vi "Catch_screw(start_side).vi"(6 "向哪校正":T1(ring)=enum."right", 7 "櫃子在哪?":enum16{"前面", "左邊", "右邊"}(ring), 8 "Error In":errorcluster) -> (0 "Error Out":errorcluster, 3 "it2(nut)":string)   [LabVIEW 2019]
uses:
  WSCbot_V3_Toolkit.lvlibp/WSCBOTV3_Toolkit/IO/LowLevel/PulseCounter.ctl
  WSCbot_V3_Toolkit.lvlibp
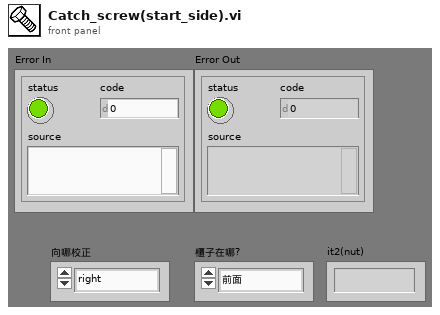
[diagram p1: front panel]
types:
  T1 = enum16{"Right_up", "Right_down", "Left_down", "Left_up", "left", "right", "up", "down"}
  T2 = typedef "WSCbot_V3_Toolkit.lvlibp/PulseCounter.ctl" = enum16{"CH1", "CH2", "CH3", "CH4", "CH5"}
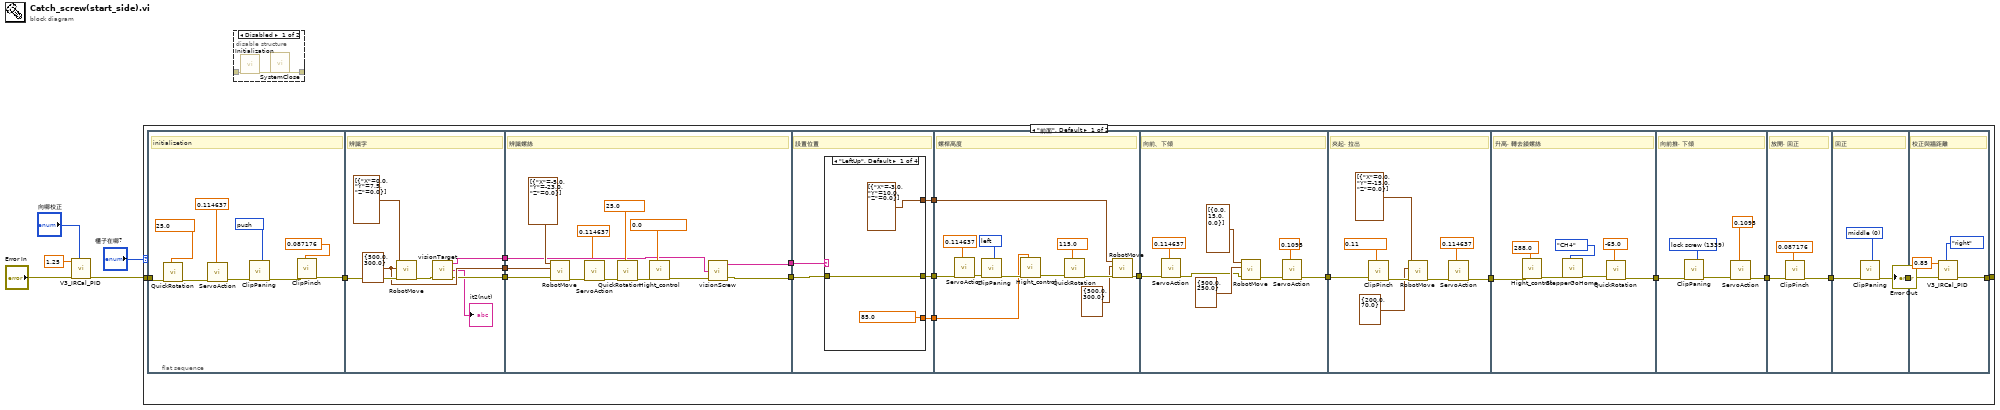
[diagram p0: block diagram]
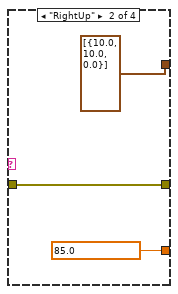
[diagram p2: hidden frame]
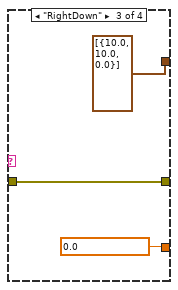
[diagram p3: hidden frame]
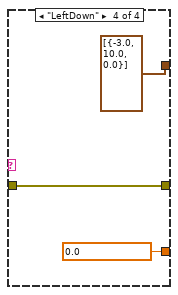
[diagram p4: hidden frame]
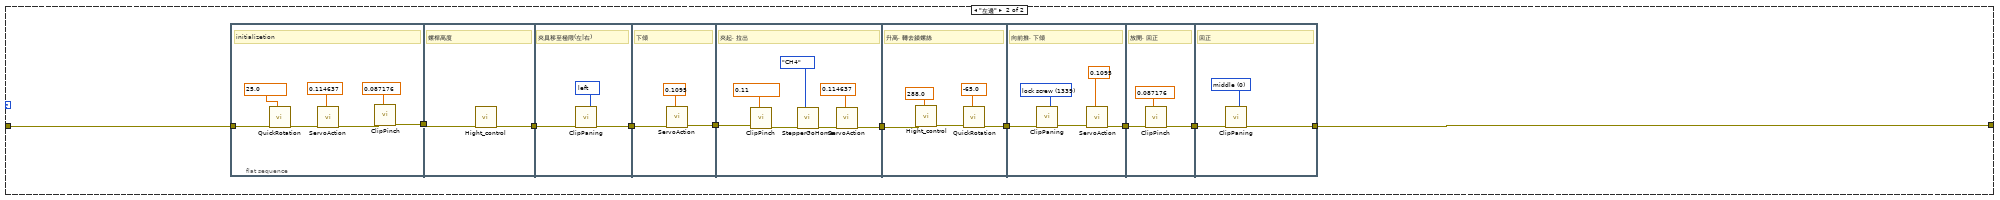
[diagram p5: hidden frame]
diagram:
  n1 = call "V3_IRCal_PID.vi"("Direction"="向哪校正", "Error In"="Error In", "X_distance(V)"=1.25) -> ("Error Out"=w4:errorcluster)  [unwired: 7 in, 1 out]
  n2 = case shown="\"前面\", Default" "櫃子在哪?" {
    tunnel: [w8 w122] -> w6
    tunnel: w4 -> [w19 w121]
    frame "前面", Default {
      n3 = flat-sequence {
        tunnel: [w28] -> w18
        tunnel: w19 -> [w27]
        tunnel: w18 -> [w39]
        tunnel: [w38] -> w17
        tunnel: [w37] -> w16
        tunnel: [w35] -> w15
        tunnel: w17 -> [w45]
        tunnel: w16 -> [w43]
        tunnel: w15 -> [w47]
        tunnel: [w44] -> w13
        tunnel: [w42] -> w12
        tunnel: w13 -> [w58]
        tunnel: w12 -> [w57]
        tunnel: [w56] -> w11
        tunnel: [w55] -> w10
        tunnel: [w54] -> w7
        tunnel: [w80] -> w14
        tunnel: w11 -> [w79]
        tunnel: w10 -> [w77]
        tunnel: w7 -> [w71]
        tunnel: [w90] -> w24
        tunnel: w14 -> [w84]
        tunnel: [w96] -> w23
        tunnel: w24 -> [w97]
        tunnel: w23 -> [w103]
        tunnel: [w104] -> w22
        tunnel: w22 -> [w110]
        tunnel: [w106] -> w21
        tunnel: w21 -> [w113]
        tunnel: [w111] -> w20
        tunnel: w20 -> [w115]
        tunnel: [w114] -> w9
        tunnel: w9 -> [w120]
        tunnel: [w119] -> w8
        frame #0 {
          w25 = 0.114637 items=["up"=0.107, "lock_up"=0.111528, "up_up"=0.114637, "down"=0.073446, "back"=0.037435, "back_back"=0.035] ("face_dir")
          w26 = -2700 items=["left"=2250, "right"=-3500, "lock screw"=1345, "lock_nut"=1167, "push"=-2700, "middle"=0] ("location")
          w32 = 25.0 items=["Forward"=25.0, "Right"=115.0, "Left"=-65.0] ("螺桿面向")
          w31 = 0.087176 items=["pinch_up"=0.11, "release"=0.087176] ("pinch?")
          # "initializetion"
          n4 = call "QuickRotation.vi"("螺桿面向"=w32, "Error In"=w27) -> ("Error Out"=w33:errorcluster)  [unwired: 9 in]
          n5 = call "ServoAction.vi"("face_dir"=w25, "Error In"=w33) -> ("Error Out"=w29:errorcluster)  [unwired: 9 in]
          n6 = call "ClipPaning.vi"("Error In"=w29, "location"=w26) -> ("Error Out"=w30:errorcluster)  [unwired: 8 in]
          n7 = call "ClipPinch.vi"("pinch?"=w31, "Error In"=w30) -> ("Error Out"=w28:errorcluster)  [unwired: 9 in]
        }
        frame #1 {
          w37 = cluster{dbl, dbl} {500.0, 300.0} ("Speed/ACC")
          # "辨識字"
          n8 = call "RobotMove.vi"("error in (no error)"=w39, "Speed/ACC"=w37, "XYZ"=cluster{"X":dbl, "Y":dbl, "Z":dbl}[] [{"X"=0.0, "Y"=7.5, "Z"=0.0}]) -> ("error out"=w36:errorcluster)  [unwired: 8 in]
          n9 = call "visionTarget.vi"("Error In"=w36) -> ("Error Out"=w35:errorcluster, "it2(nut)"=→"it2(nut)":string, "it1(screw)"=w38:string)  [unwired: 2 in]
        }
        frame #2 {
          w41 = 0.114637 items=["up"=0.107, "lock_up"=0.111528, "up_up"=0.114637, "down"=0.073446, "back"=0.037435, "back_back"=0.035] ("face_dir")
          w48 = 0.0 items=["物料櫃第一格"=0.0, "物料櫃第二格"=78.0, "螺帽夾取高度"=128.0, "螺帽瞄準"=250.0, "最高"=288.0] ("螺桿高度")
          w50 = 25.0 items=["Forward"=25.0, "Right"=115.0, "Left"=-65.0] ("螺桿面向")
          # "辨識螺絲"
          n10 = call "RobotMove.vi"("error in (no error)"=w47, "Speed/ACC"=w43, "XYZ"=cluster{"X":dbl, "Y":dbl, "Z":dbl}[] [{"X"=-5.0, "Y"=-23.0, "Z"=0.0}]) -> ("error out"=w52:errorcluster)  [unwired: 8 in]
          n11 = call "ServoAction.vi"("face_dir"=w41, "Error In"=w52) -> ("Error Out"=w51:errorcluster)  [unwired: 9 in]
          n12 = call "QuickRotation.vi"("螺桿面向"=w50, "Error In"=w51) -> ("Error Out"=w49:errorcluster)  [unwired: 9 in]
          n13 = call "Hight_control.vi"("螺桿高度"=w48, "Error In"=w49) -> ("Error Out"=w46:errorcluster)  [unwired: 9 in]
          n14 = call "visionScrew.vi"("Error In"=w46, "Aim_Color"=w45) -> ("Error Out"=w42:errorcluster, "Position"=w44:string)  [unwired: 2 in]
        }
        frame #3 {
          # "設置位置"
          n15 = case shown="\"LeftUp\", Default" w58 {
            tunnel: w57 -> [w60 w63 w66 w69]
            tunnel: [cluster{"X":dbl, "Y":dbl, "Z":dbl}[] [{"X"=-3.0, "Y"=10.0, "Z"=0.0}] ("XYZ") cluster{"X":dbl, "Y":dbl, "Z":dbl}[] [{"X"=10.0, "Y"=10.0, "Z"=0.0}] ("XYZ") cluster{"X":dbl, "Y":dbl, "Z":dbl}[] [{"X"=10.0, "Y"=10.0, "Z"=0.0}] ("XYZ") cluster{"X":dbl, "Y":dbl, "Z":dbl}[] [{"X"=-3.0, "Y"=10.0, "Z"=0.0}] ("XYZ")] -> w56
            tunnel: [w60 w63 w66 w69] -> w55
            tunnel: [w59 w62 w65 w68] -> w54
            frame "LeftUp", Default {
              w59 = 85.0 items=["物料櫃第一格"=0.0, "物料櫃第二格"=85.0, "螺帽夾取高度"=128.0, "螺帽瞄準"=250.0, "最高"=288.0] ("螺桿高度")
            }
            frame "RightUp" {
              w62 = 85.0 items=["物料櫃第一格"=0.0, "物料櫃第二格"=85.0, "螺帽夾取高度"=128.0, "螺帽瞄準"=250.0, "最高"=288.0] ("螺桿高度")
            }
            frame "RightDown" {
              w65 = 0.0 items=["物料櫃第一格"=0.0, "物料櫃第二格"=85.0, "螺帽夾取高度"=128.0, "螺帽瞄準"=250.0, "最高"=288.0] ("螺桿高度")
            }
            frame "LeftDown" {
              w68 = 0.0 items=["物料櫃第一格"=0.0, "物料櫃第二格"=85.0, "螺帽夾取高度"=128.0, "螺帽瞄準"=250.0, "最高"=288.0] ("螺桿高度")
            }
          }
        }
        frame #4 {
          w72 = 0.114637 items=["up"=0.107, "lock_up"=0.111528, "up_up"=0.114637, "down"=0.073446, "back"=0.037435, "back_back"=0.035] ("face_dir")
          w82 = 2100 items=["left"=2100, "right"=-3500, "lock screw"=1345, "lock_nut"=1167, "middle"=0] ("location")
          w75 = 115.0 items=["Forward"=25.0, "Right"=115.0, "Left"=-65.0] ("螺桿面向")
          # "螺桿高度"
          n16 = call "ServoAction.vi"("face_dir"=w72, "Error In"=w77) -> ("Error Out"=w76:errorcluster)  [unwired: 9 in]
          n17 = call "ClipPaning.vi"("Error In"=w76, "location"=w82) -> ("Error Out"=w74:errorcluster)  [unwired: 8 in]
          n18 = call "Hight_control.vi"("螺桿高度"=w71, "Error In"=w74) -> ("Error Out"=w73:errorcluster)  [unwired: 9 in]
          n19 = call "QuickRotation.vi"("螺桿面向"=w75, "Error In"=w73) -> ("Error Out"=w81:errorcluster)  [unwired: 9 in]
          n20 = call "RobotMove.vi"("error in (no error)"=w81, "Speed/ACC"=cluster{dbl, dbl} {500.0, 300.0}, "XYZ"=w79) -> ("error out"=w80:errorcluster)  [unwired: 8 in]
        }
        frame #5 {
          w85 = 0.114637 items=["up"=0.1095, "up_up"=0.114637, "down"=0.073446, "back"=0.037435, "back_back"=0.035] ("face_dir")
          w89 = 0.1095 items=["up"=0.1095, "up_up"=0.114637, "down"=0.073446, "back"=0.037435, "back_back"=0.035] ("face_dir")
          # "向前、下傾"
          n21 = call "ServoAction.vi"("face_dir"=w85, "Error In"=w84) -> ("Error Out"=w83:errorcluster)  [unwired: 9 in]
          n22 = call "RobotMove.vi"("error in (no error)"=w83, "Speed/ACC"=cluster{dbl, dbl} {500.0, 250.0}, "XYZ"=cluster{"X":dbl, "Y":dbl, "Z":dbl}[] [{"X"=0.0, "Y"=15.0, "Z"=0.0}]) -> ("error out"=w88:errorcluster)  [unwired: 8 in]
          n23 = call "ServoAction.vi"("face_dir"=w89, "Error In"=w88) -> ("Error Out"=w90:errorcluster)  [unwired: 9 in]
        }
        frame #6 {
          w95 = 0.114637 items=["up"=0.1095, "up_up"=0.114637, "down"=0.073446, "back"=0.037435, "back_back"=0.035] ("face_dir")
          w98 = 0.11 items=["pinch_up"=0.11, "release"=0.087176] ("pinch?")
          # "夾起, 拉出"
          n24 = call "ClipPinch.vi"("pinch?"=w98, "Error In"=w97) -> ("Error Out"=w94:errorcluster)  [unwired: 9 in]
          n25 = call "RobotMove.vi"("error in (no error)"=w94, "Speed/ACC"=cluster{dbl, dbl} {200.0, 70.0}, "XYZ"=cluster{"X":dbl, "Y":dbl, "Z":dbl}[] [{"X"=0.0, "Y"=-15.0, "Z"=0.0}]) -> ("error out"=w93:errorcluster)  [unwired: 8 in]
          n26 = call "ServoAction.vi"("face_dir"=w95, "Error In"=w93) -> ("Error Out"=w96:errorcluster)  [unwired: 9 in]
        }
        frame #7 {
          w102 = 288.0 items=["物料櫃第一格"=0.0, "物料櫃第二格"=78.0, "螺帽夾取高度"=128.0, "螺帽瞄準"=250.0, "最高"=288.0] ("螺桿高度")
          w105 = -65.0 items=["Forward"=25.0, "Right"=115.0, "Left"=-65.0] ("螺桿面向")
          # "升高, 轉去鎖螺絲"
          n27 = call "Hight_control.vi"("螺桿高度"=w102, "Error In"=w103) -> ("Error Out"=w100:errorcluster)  [unwired: 9 in]
          n28 = call "StepperGoHome.vi"("PulseCounterChanel"=PulseCounter."CH4", "Error In"=w100) -> ("Error Out"=w99:errorcluster)  [unwired: 7 in, 2 out]
          n29 = call "QuickRotation.vi"("螺桿面向"=w105, "Error In"=w99) -> ("Error Out"=w104:errorcluster)  [unwired: 9 in]
        }
        frame #8 {
          w107 = 0.1095 items=["up"=0.1095, "up_up"=0.114637, "down"=0.073446, "back"=0.037435, "back_back"=0.035] ("face_dir")
          w109 = 1339 items=["left"=2100, "right"=-3500, "lock screw"=1339, "middle"=0] ("location")
          # "向前推, 下傾"
          n30 = call "ClipPaning.vi"("Error In"=w110, "location"=w109) -> ("Error Out"=w108:errorcluster)  [unwired: 8 in]
          n31 = call "ServoAction.vi"("face_dir"=w107, "Error In"=w108) -> ("Error Out"=w106:errorcluster)  [unwired: 9 in]
        }
        frame #9 {
          w112 = 0.087176 items=["pinch_up"=0.11, "release"=0.087176] ("pinch?")
          # "放開, 回正"
          n32 = call "ClipPinch.vi"("pinch?"=w112, "Error In"=w113) -> ("Error Out"=w111:errorcluster)  [unwired: 9 in]
        }
        frame #10 {
          w116 = 0 items=["left"=2100, "right"=-3500, "lock screw"=1339, "middle"=0] ("location")
          # "回正"
          n33 = call "ClipPaning.vi"("Error In"=w115, "location"=w116) -> ("Error Out"=w114:errorcluster)  [unwired: 8 in]
        }
        frame #11 {
          # "校正與牆距離"
          n34 = call "V3_IRCal_PID.vi"("Direction"=T1."right", "Error In"=w120, "X_distance(V)"=0.85) -> ("Error Out"=w119:errorcluster)  [unwired: 7 in, 1 out]
        }
      }
    }
    frame "左邊" {
      n35 = flat-sequence {
        tunnel: [w134] -> w130
        tunnel: w121 -> [w132]
        tunnel: w130 -> [w139]
        tunnel: [w138] -> w129
        tunnel: [w142] -> w128
        tunnel: w129 -> [w140]
        tunnel: w128 -> [w144]
        tunnel: [w145] -> w127
        tunnel: [w147] -> w126
        tunnel: w127 -> [w149]
        tunnel: w126 -> [w155]
        tunnel: [w156] -> w125
        tunnel: w125 -> [w162]
        tunnel: [w158] -> w124
        tunnel: w124 -> [w165]
        tunnel: [w163] -> w123
        tunnel: w123 -> [w167]
        tunnel: [w166] -> w122
        frame #0 {
          w131 = 25.0 items=["Forward"=25.0, "Right"=115.0, "Left"=-65.0] ("螺桿面向")
          w136 = 0.087176 items=["pinch_up"=0.11, "release"=0.087176] ("pinch?")
          w137 = 0.114637 items=["up"=0.1095, "up_up"=0.114637, "down"=0.073446, "back"=0.037435, "back_back"=0.035] ("face_dir")
          # "initializetion"
          n36 = call "QuickRotation.vi"("螺桿面向"=w131, "Error In"=w132) -> ("Error Out"=w133:errorcluster)  [unwired: 9 in]
          n37 = call "ServoAction.vi"("face_dir"=w137, "Error In"=w133) -> ("Error Out"=w135:errorcluster)  [unwired: 9 in]
          n38 = call "ClipPinch.vi"("pinch?"=w136, "Error In"=w135) -> ("Error Out"=w134:errorcluster)  [unwired: 9 in]
        }
        frame #1 {
          # "螺桿高度"
          n39 = call "Hight_control.vi"("Error In"=w139) -> ("Error Out"=w138:errorcluster)  [unwired: 10 in]
        }
        frame #2 {
          w141 = 2100 items=["left"=2100, "right"=-3500, "lock screw"=1339, "middle"=0] ("location")
          # "夾具移至極限(左|右)"
          n40 = call "ClipPaning.vi"("Error In"=w140, "location"=w141) -> ("Error Out"=w142:errorcluster)  [unwired: 8 in]
        }
        frame #3 {
          w143 = 0.1095 items=["up"=0.1095, "up_up"=0.114637, "down"=0.073446, "back"=0.037435, "back_back"=0.035] ("face_dir")
          # "下傾"
          n41 = call "ServoAction.vi"("face_dir"=w143, "Error In"=w144) -> ("Error Out"=w145:errorcluster)  [unwired: 9 in]
        }
        frame #4 {
          w146 = 0.114637 items=["up"=0.1095, "up_up"=0.114637, "down"=0.073446, "back"=0.037435, "back_back"=0.035] ("face_dir")
          w152 = 0.11 items=["pinch_up"=0.11, "release"=0.087176] ("pinch?")
          # "夾起, 拉出"
          n42 = call "ClipPinch.vi"("pinch?"=w152, "Error In"=w149) -> ("Error Out"=w151:errorcluster)  [unwired: 9 in]
          n43 = call "StepperGoHome.vi"("PulseCounterChanel"=PulseCounter."CH4", "Error In"=w151) -> ("Error Out"=w148:errorcluster)  [unwired: 7 in, 2 out]
          n44 = call "ServoAction.vi"("face_dir"=w146, "Error In"=w148) -> ("Error Out"=w147:errorcluster)  [unwired: 9 in]
        }
        frame #5 {
          w153 = 288.0 items=["物料櫃第一格"=0.0, "物料櫃第二格"=78.0, "螺帽夾取高度"=128.0, "螺帽瞄準"=250.0, "最高"=288.0] ("螺桿高度")
          w157 = -65.0 items=["Forward"=25.0, "Right"=115.0, "Left"=-65.0] ("螺桿面向")
          # "升高, 轉去鎖螺絲"
          n45 = call "Hight_control.vi"("螺桿高度"=w153, "Error In"=w155) -> ("Error Out"=w154:errorcluster)  [unwired: 9 in]
          n46 = call "QuickRotation.vi"("螺桿面向"=w157, "Error In"=w154) -> ("Error Out"=w156:errorcluster)  [unwired: 9 in]
        }
        frame #6 {
          w159 = 0.1095 items=["up"=0.1095, "up_up"=0.114637, "down"=0.073446, "back"=0.037435, "back_back"=0.035] ("face_dir")
          w161 = 1339 items=["left"=2100, "right"=-3500, "lock screw"=1339, "middle"=0] ("location")
          # "向前推, 下傾"
          n47 = call "ClipPaning.vi"("Error In"=w162, "location"=w161) -> ("Error Out"=w160:errorcluster)  [unwired: 8 in]
          n48 = call "ServoAction.vi"("face_dir"=w159, "Error In"=w160) -> ("Error Out"=w158:errorcluster)  [unwired: 9 in]
        }
        frame #7 {
          w164 = 0.087176 items=["pinch_up"=0.11, "release"=0.087176] ("pinch?")
          # "放開, 回正"
          n49 = call "ClipPinch.vi"("pinch?"=w164, "Error In"=w165) -> ("Error Out"=w163:errorcluster)  [unwired: 9 in]
        }
        frame #8 {
          w168 = 0 items=["left"=2100, "right"=-3500, "lock screw"=1339, "middle"=0] ("location")
          # "回正"
          n50 = call "ClipPaning.vi"("Error In"=w167, "location"=w168) -> ("Error Out"=w166:errorcluster)  [unwired: 8 in]
        }
      }
    }
  }
  "Error Out" <- w6
  n51 = disable-structure shown="Disabled" {
    disable-tunnel: [w170 _] -> _
    disable-tunnel: _ -> [w169 _]
    frame Disabled {
      n52 = call "Initialization.vi"("Error In"=w169) -> ("Error Out"=w170:errorcluster)  [unwired: 10 in]
      n53 = call "SystemClose.vi"() -> ()  [unwired: 3 in, 1 out]
    }
    frame Enabled {
    }
  }
